vi "Simple_Example_Soft_Trigger.vi"() -> ()   [LabVIEW 2019]
doc: "This example shows a simple recording of an image sequence and the image access afterwards.\nIt is a good starting point for writing own applications.\nBut it will not be fail save, i.e. doesnt react on errors, just handles them forward to the end\n\nUsage:\nSelect your required image count before you start the program. Press the \"Trigger\" button to acquire an image. Once started, the camera class will be initialized and images will be recorded automatically.\nWhen acquisition has finished you can address the images and set a certain roi \nTo finish the program click on quit application, this will force fan exit of the camera class"
uses:
  camera/Camera.lvclass
  <vilib>/picture/picture.llb/Draw 8-Bit Pixmap.vi
  <vilib>/picture/picture.llb/Draw True-Color Pixmap.vi
  pco.sdk/TimingControl/TimingControl.lvlib
panel:
  in  "Trigger":bool
  out "colormap(U8)":u32[](array[numeric])
  out "Image(U16)":u16[][](graph)
  in  "Zoom [%]":i32(slide)=26 min=10 max=200 step=5 scale=10.0..200.0
  out "Image":picture
  out "rawImage":u16[][](array[numeric])
  in  "data_format":T1(ring)=enum."Mono16"
  in  "Image Index":u32 max=9
  out "Recorded Images":u32
  in  "Quit":bool
  in  "cropY1":u64=2 min=2 max=2048 step=1
  in  "cropX1":u64=2 min=2 max=2048 step=1
  in  "cropY0":u64=1 min=1 max=2047 step=1
  in  "cropX0":u64=1 min=1 max=2047 step=1
  out "Image Height":u16
  out "Image Width":u16
  in  "dwImgCount":u32=10 caption="Required Number of Images" max=4023
  out "Error":errorcluster {"code" format="%x"}
  # "This example shows a simple recording of an image sequence using software triggering and the image access afterwards.\nIt is a good starting point for writing own applications.\nBut it will not be fail save, i.e. doesnt react on errors, just handles them forward to the end\n\nUsage:\nSelect your required image count before you start the program. Once started, the camera class will be initialized and images will be recorded automatically. Press the \"Trigger\" button to acquire an image. When acquisition has finished you can address the images and crop them to a smaller size. To finish the program click on quit application, this will force fan exit of the camera class"
  # "pco.labview"
  # "Camera Setup"
  # "Recording Control"
  # "Parameters for image readout"
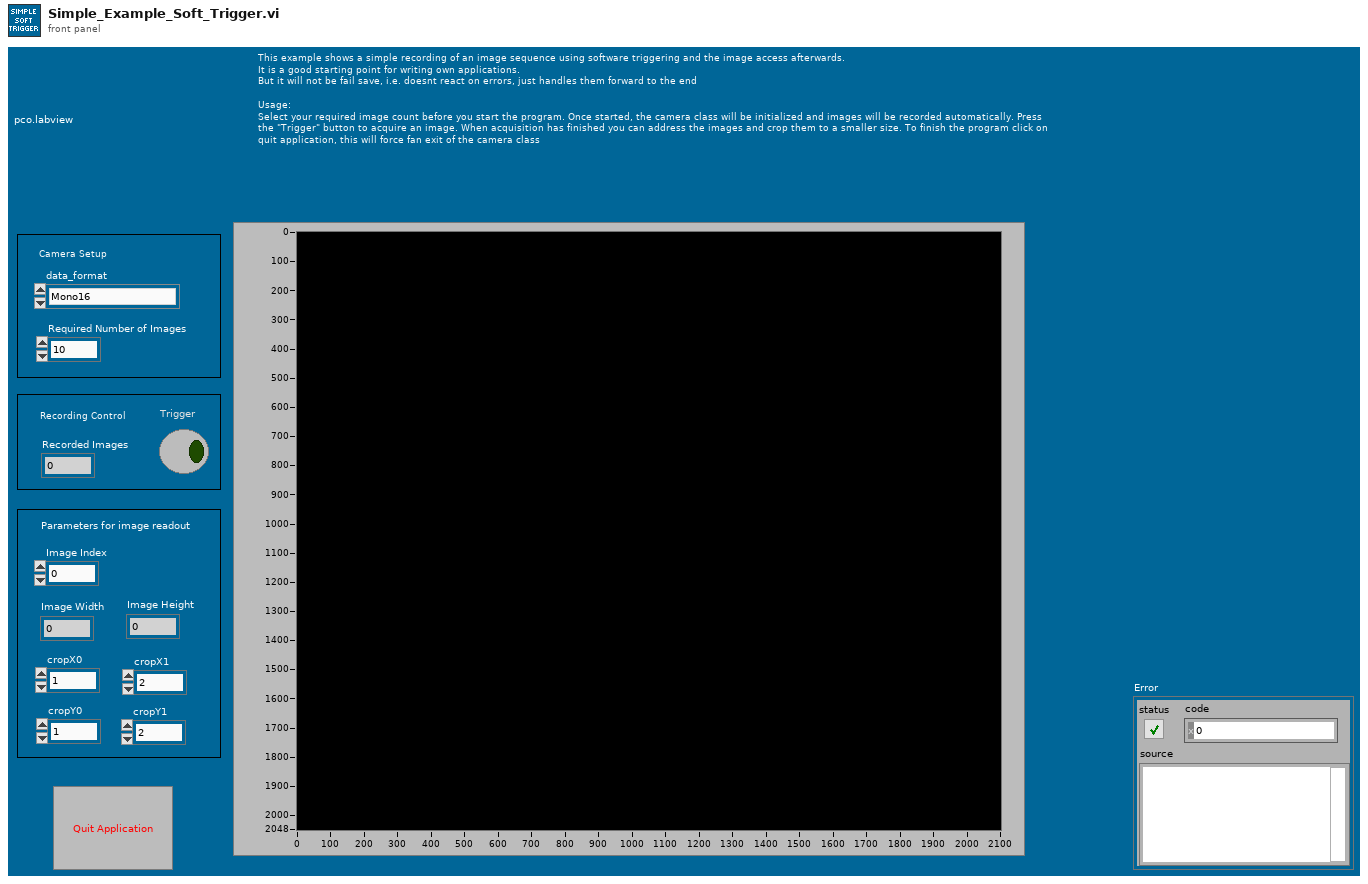
[diagram p1: front panel]
types:
  T1 = enum16{"Undefined", "Mono8", "Mono16", "BGRA8", "RGBA8", "BGRA16", "RGBA16", "CompressedMono8"}
  T2 = enum8{"Enabled", "Disabled", "Disabled and Grayed Out"}
  T3 = enum16{"sequence", "sequence non blocking", "ring buffer", "fifo", "tif", "multitif", "pcoraw", "b16", "dicom", "multidicom", "camram_ring", "camram_segment"}
  T4 = typedef "Camera.lvclass/binning.ctl" = cluster{"vert":u16, "horz":u16, "mode":u16}
  T5 = cluster{"exposure_time_s":dbl, "delay_time_s":dbl, "roi":cluster{"x0":u64, "y0":u64, "x1":u64, "y1":u64}, "timestamp_mode":u16, "pixelrate":u32, "conversion_factor":sgl, "trigger_mode":u16, "acquire_mode":u16, "acquire_sequence_number":u32, "metadata_mode":u16, "noisefilter_mode":u16, "pixel_format":u32, "binning":T4, "auto_exposure":cluster{"region":u16, "min_exposure_s":dbl, "max_exposure_s":dbl}}
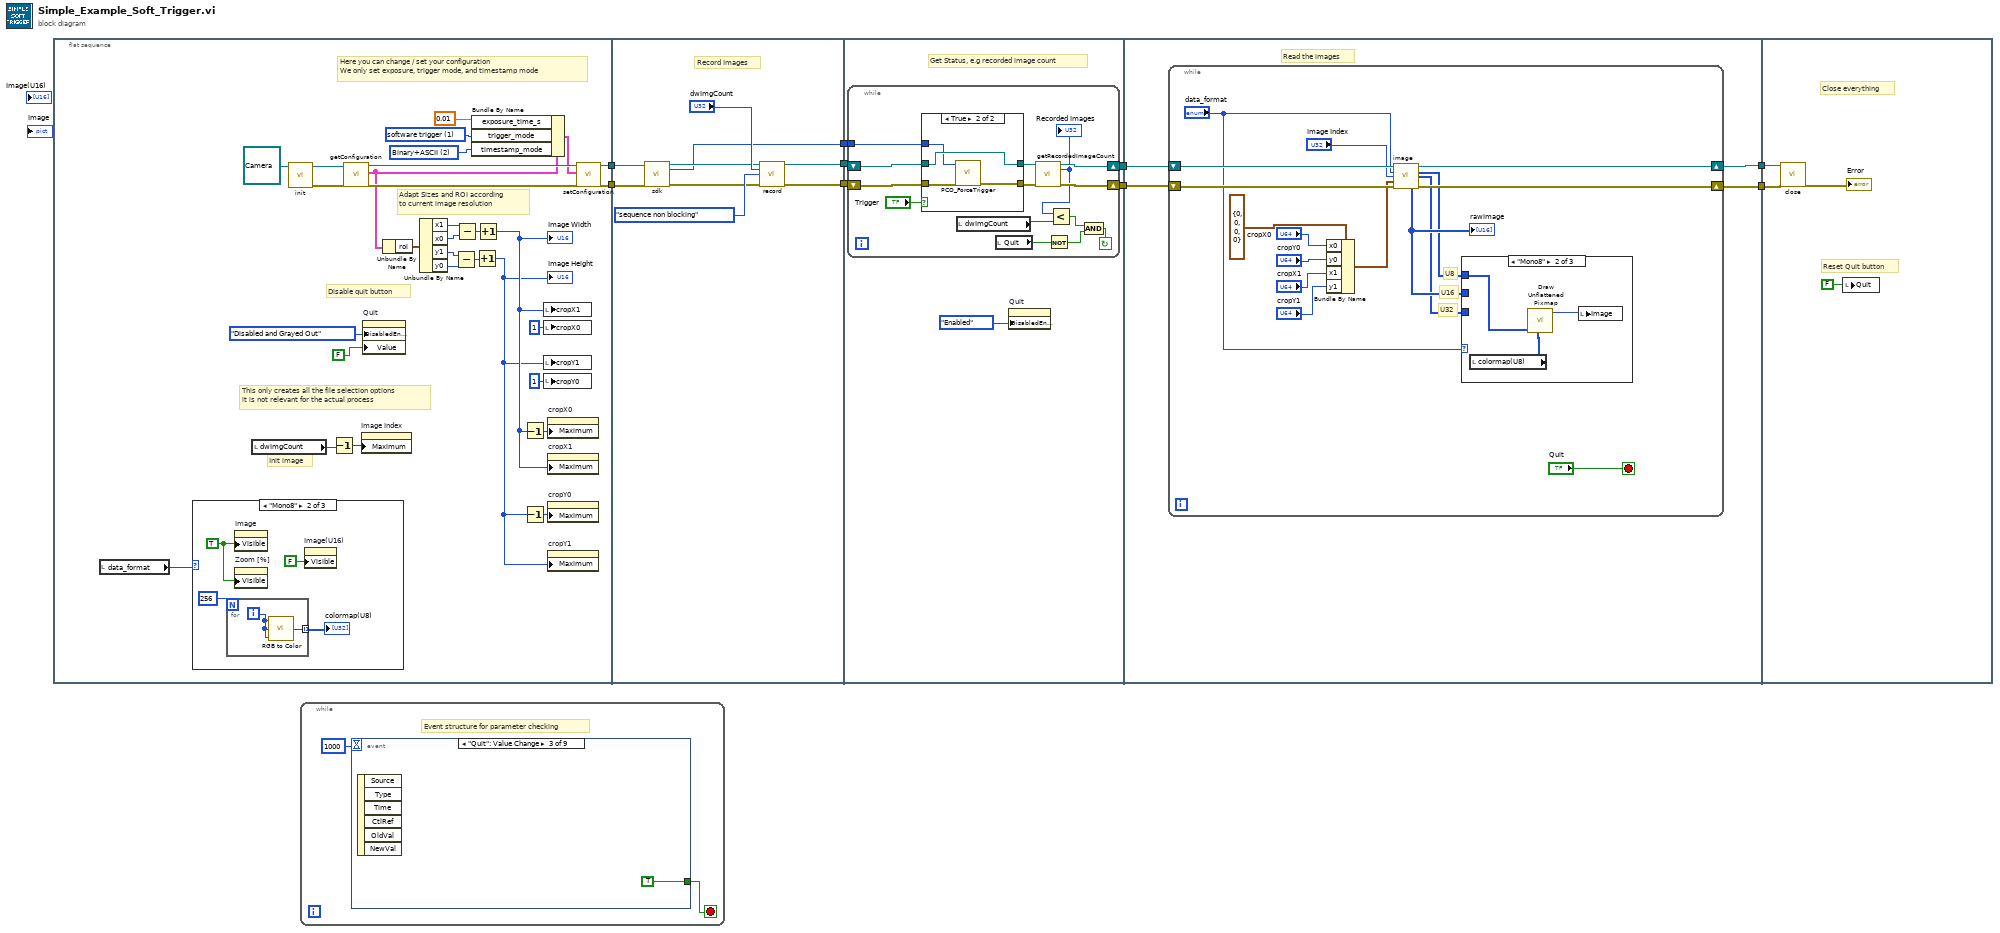
[diagram p0: block diagram]
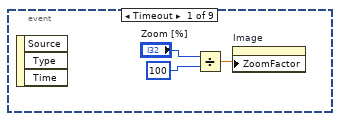
[diagram p2: hidden frame]
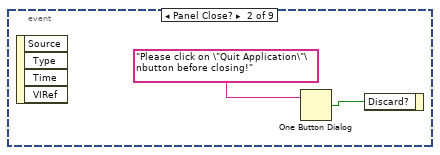
[diagram p3: hidden frame]
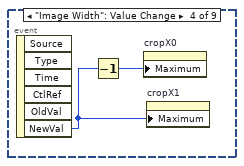
[diagram p4: hidden frame]
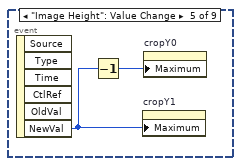
[diagram p5: hidden frame]
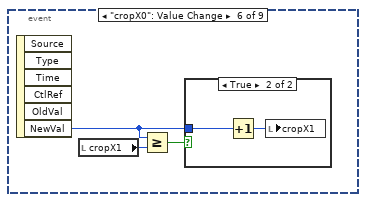
[diagram p6: hidden frame]
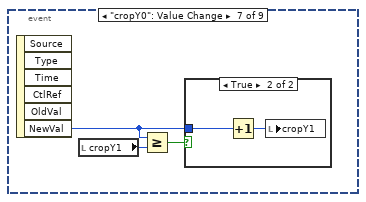
[diagram p8: hidden frame]
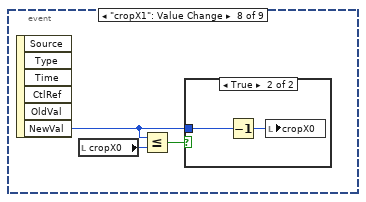
[diagram p10: hidden frame]
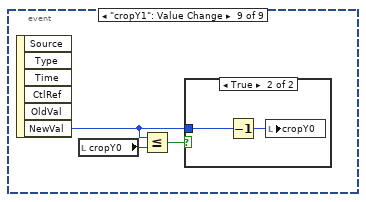
[diagram p12: hidden frame]
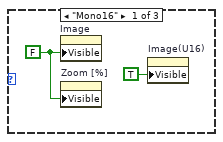
[diagram p14: hidden frame]
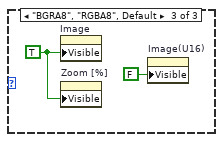
[diagram p15: hidden frame]
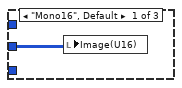
[diagram p17: hidden frame]
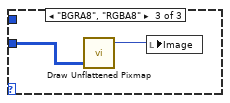
[diagram p18: hidden frame]
diagram:
  n1 = flat-sequence {
    tunnel: [w32] -> w9
    tunnel: [w31] -> w8
    tunnel: w9 -> [w54]
    tunnel: w8 -> [w52]
    tunnel: [w57] -> w7
    tunnel: [w56] -> w6
    tunnel: [w50] -> w1
    tunnel: w7 -> [w61]
    tunnel: w6 -> [w60]
    tunnel: [w64] -> w5
    tunnel: [w63] -> w4
    tunnel: w1 -> [w59]
    tunnel: w5 -> [w87]
    tunnel: w4 -> [w88]
    tunnel: [w86] -> w3
    tunnel: [w85] -> w2
    tunnel: w3 -> [w112]
    tunnel: w2 -> [w111]
    frame #0 {
      w16 = u16 2 items=["OFF", "Binary", "Binary+ASCII", "ASCII"] ("TimestampMode")
      w36 = u16 1 items=["auto sequence"=0, "software trigger"=1, "external exposure start & software trigger"=2, "external exposure control"=3, "external synchronized"=4, "fast external exposure control"=5, "external CDS control"=6, "slow external exposure control"=7, "external synchronized HDSDI"=258] ("TriggerMode")
      # "Here you can change / set your configuration\nWe only set exposure, trigger mode, and timestamp mode"
      # "Init image"
      # "This only creates all the file selection options\nit is not relevant for the actual process"
      # "Adapt Sizes and ROI according\nto current image resolution"
      # "Disable quit button"
      n2 = local read "data_format"() -> (w11:T1)
      n3 = case shown="\"Mono8\"" w11 {
        frame "Mono16" {
          w41 = FALSE ("Visible")
          n4 = property on="Image" class="Pict"("Visible"=w41) -> ()  [unwired: 2 in, 2 out]
          n5 = property on="Zoom [%]" class="Slide (strict)"("Visible"=w41) -> ()  [unwired: 2 in, 2 out]
          n6 = property on="Image(U16)" class="IntGraph (strict)"("Visible"=TRUE) -> ()  [unwired: 2 in, 2 out]
        }
        frame "Mono8" {
          w44 = TRUE ("Visible")
          n7 = for {
            N: 256 -> [_]
            tunnel: [w46] -> w43 mode=indexing
            i -> [w47]
            n8 = call <vilib>:"RGB to Color.vi"("B"=w47, "G"=w47, "R"=w47) -> ("Color"=w46:u32)
          }
          "colormap(U8)" <- w43
          n9 = property on="Image" class="Pict"("Visible"=w44) -> ()  [unwired: 2 in, 2 out]
          n10 = property on="Zoom [%]" class="Slide (strict)"("Visible"=w44) -> ()  [unwired: 2 in, 2 out]
          n11 = property on="Image(U16)" class="IntGraph (strict)"("Visible"=FALSE) -> ()  [unwired: 2 in, 2 out]
        }
        frame "BGRA8", "RGBA8", Default {
          w48 = TRUE ("Visible")
          n12 = property on="Image" class="Pict"("Visible"=w48) -> ()  [unwired: 2 in, 2 out]
          n13 = property on="Zoom [%]" class="Slide (strict)"("Visible"=w48) -> ()  [unwired: 2 in, 2 out]
          n14 = property on="Image(U16)" class="IntGraph (strict)"("Visible"=FALSE) -> ()  [unwired: 2 in, 2 out]
        }
      }
      n15 = local read "dwImgCount"() -> (w12:u32)
      n16 = call-dynamic "init.vi"("Camera in"=refnum<class "Camera.lvclass"> refnum ("PCOCamera in")) -> ("Camera out"=w38:refnum<class "Camera.lvclass">, "error out"=w37:errorcluster)  [unwired: 8 in]
      n17 = Decrement(x=w12) -> (x-1=w13:u32)
      n18 = call-dynamic "getConfiguration.vi"("error in (no error)"=w37, "Camera in"=w38) -> ("error out"=w34:errorcluster, "configuration"=w26:T5, "Camera out"=w35:refnum<class "Camera.lvclass">)  [unwired: 7 in]
      n19 = property on="Image Index" class="DigNum (strict)"("Maximum"=w13) -> ()  [unwired: 2 in, 2 out]
      n20 = property on="Quit" class="Bool (strict)"("DisabledEnum"=T2."Disabled and Grayed Out" ("Disabled"), "Value"=FALSE ("Stop")) -> ()  [unwired: 2 in, 2 out]
      n21 = Unbundle By Name(w26) -> ("roi"=w25:cluster{"x0":u64, "y0":u64, "x1":u64, "y1":u64})
      n22 = Unbundle By Name(w25) -> ("x1"=w23:u64, "x0"=w24:u64, "y1"=w21:u64, "y0"=w22:u64)
      n23 = Subtract(x=w21, y=w22) -> (x-y=w19:u64)
      n24 = Subtract(x=w23, y=w24) -> (x-y=w20:u64)
      n25 = Bundle By Name(cluster=w26, "exposure_time_s"=0.01, "trigger_mode"=w36, "timestamp_mode"=w16) -> (w33:T5)
      n26 = Increment(x=w19) -> (x+1=w17:u64)
      "Image Height" <- w17
      n27 = Increment(x=w20) -> (x+1=w18:u64)
      "Image Width" <- w18
      n28 = Decrement(x=w18) -> (x-1=w28:u64)
      n29 = Decrement(x=w17) -> (x-1=w27:u64)
      n30 = local write "cropX1"(w18) -> ()
      n31 = local write "cropX0"(u16 1 ("roiY0")) -> ()
      n32 = local write "cropY1"(w17) -> ()
      n33 = local write "cropY0"(u16 1 ("roiY0")) -> ()
      n34 = property on="cropX0" class="DigNum (strict)"("Maximum"=w28) -> ()  [unwired: 2 in, 2 out]
      n35 = property on="cropX1" class="DigNum (strict)"("Maximum"=w18) -> ()  [unwired: 2 in, 2 out]
      n36 = property on="cropY0" class="DigNum (strict)"("Maximum"=w27) -> ()  [unwired: 2 in, 2 out]
      n37 = property on="cropY1" class="DigNum (strict)"("Maximum"=w17) -> ()  [unwired: 2 in, 2 out]
      n38 = call-dynamic "setConfiguration.vi"("error in (no error)"=w34, "configuration"=w33, "Camera in"=w35) -> ("error out"=w31:errorcluster, "Camera out"=w32:refnum<class "Camera.lvclass">)  [unwired: 7 in]
    }
    frame #1 {
      # "Record Images"
      n39 = call-dynamic "sdk.vi"("Camera in"=w54, "error in (no error)"=w52) -> ("Camera out"=w53:refnum<class "Camera.lvclass">, "sdk"=w50:u64, "error out"=w51:errorcluster)  [unwired: 11 in]
      n40 = call-dynamic "record.vi"("Camera in"=w53, "num_images"="dwImgCount", "record_mode"=T3."sequence non blocking", "error in (no error)"=w51) -> ("Camera out"=w57:refnum<class "Camera.lvclass">, "error out"=w56:errorcluster)  [unwired: 10 in]
    }
    frame #2 {
      # "Get Status, e.g recorded image count"
      n41 = while {
        tunnel: w59 -> [w72]
        shift-right: [w78] -> w64
        shift-left: w61 -> [w76]
        shift-right: [w77] -> w63
        shift-left: w60 -> [w74]
        stop <- w65 continue-if-true
        n42 = case shown="True" "Trigger" {
          tunnel: w76 -> [w80 w84]
          tunnel: [w80 w84] -> w75
          tunnel: w74 -> [w79 w83]
          tunnel: [w79 w82] -> w73
          tunnel: w72 -> [_ w81]
          frame False {
          }
          frame True {
            n43 = call "PCO_ForceTrigger.vi"("error in (no error)"=w83, "ph"=w81) -> ("error out"=w82:errorcluster)  [unwired: 6 in, 3 out]
          }
        }
        n44 = local read "dwImgCount"() -> (w70:u32)
        n45 = local read "Quit"() -> (w68:bool)
        n46 = call-dynamic "getRecordedImageCount.vi"("Camera in"=w75, "error in (no error)"=w73) -> ("Camera out"=w78:refnum<class "Camera.lvclass">, "recorded_image_count"=w69:u32, "error out"=w77:errorcluster)  [unwired: 11 in]
        "Recorded Images" <- w69
        n47 = Not(x=w68) -> (.not. x?=w67:bool)
        n48 = Less?(x=w69, y=w70) -> (x < y?=w66:bool)
        n49 = And(x=w66, y=w67) -> (x .and. y?=w65:bool)
      }
      n50 = property on="Quit" class="Bool (strict)"("DisabledEnum"=T2."Enabled" ("Disabled")) -> ()  [unwired: 2 in, 2 out]
    }
    frame #3 {
      # "Read the images"
      n51 = while {
        shift-right: [w102] -> w86
        shift-left: w87 -> [w104]
        shift-right: [w97] -> w85
        shift-left: w88 -> [w103]
        stop <- "Quit" stop-if-true
        # "U32"
        # "U16"
        # "U8"
        n52 = Bundle By Name(cluster=cluster{"x0":u64, "y0":u64, "x1":u64, "y1":u64} {"x0"=0, "y0"=0, "x1"=0, "y1"=0} ("roi"), "x0"="cropX0", "y0"="cropY0", "x1"="cropX1", "y1"="cropY1") -> (w96:cluster{"x0":u64, "y0":u64, "x1":u64, "y1":u64})
        n53 = call-dynamic "image.vi"("Camera in"=w104, "data_format"="data_format", "image_index"="Image Index", "crop"=w96, "error in (no error)"=w103) -> ("Camera out"=w102:refnum<class "Camera.lvclass">, "image (U8)"=w89:u8[][], "image (U32)"=w90:u32[][], "raw_image (U16)"=w91:u16[][], "error out"=w97:errorcluster)  [unwired: 2 in, 4 out]
        "rawImage" <- w91
        n54 = case shown="\"Mono8\"" "data_format" {
          tunnel: w90 -> [_ _ w110]
          tunnel: w89 -> [_ w107 _]
          tunnel: w91 -> [w105 _ _]
          frame "Mono16", Default {
            n55 = local write "Image(U16)"(w105) -> ()
          }
          frame "Mono8" {
            n56 = local read "colormap(U8)"() -> (w106:u32[])
            n57 = call-poly <vilib>:"Draw Unflattened Pixmap.vi"("data"=w107, "color table"=w106) -> ("new picture"=w108:picture)  [unwired: 7 in]
            n58 = local write "Image"(w108) -> ()
          }
          frame "BGRA8", "RGBA8" {
            n59 = call-poly <vilib>:"Draw Unflattened Pixmap.vi"("data (RGB format)"=w110) -> ("new picture"=w109:picture)  [unwired: 8 in]
            n60 = local write "Image"(w109) -> ()
          }
        }
      }
    }
    frame #4 {
      # "Reset Quit button"
      # "Close everything"
      n61 = call-dynamic "close.vi"("error in (no error)"=w111, "Camera in"=w112) -> ("error out"=→"Error":errorcluster)  [unwired: 9 in]
      n62 = local write "Quit"(FALSE ("Stop")) -> ()
    }
  }
  n63 = while {
    stop <- w115 stop-if-true
    # "Event structure for parameter checking"
    n64 = event shown="[2] \"Quit\": Value Change" {
      selector: _ -> [_ _ _ _ _ _ _ _ _]
      dyn-events: _ -> [_ _ _ _ _ _ _ _ _]
      timeout: 1000 -> [_ _ _ _ _ _ _ _ _]
      tunnel: [_ _ TRUE _ _ _ _ _ _] -> w115
      event Timeout {
        n65 = event-data() -> ()  [unwired: 1 in, 3 out]
        n66 = Divide(x="Zoom [%]", y=100 ("Zoom [%]")) -> (x/y=w117:dbl)
        n67 = property on="Image" class="Pict"("ZoomFactor"=w117) -> ()  [unwired: 2 in, 2 out]
      }
      event Panel Close? {
        n68 = event-data() -> ()  [unwired: 1 in, 4 out]
        n69 = One Button Dialog(message="Please click on \"Quit Application\"\nbutton before closing!") -> (true=w120:bool)  [unwired: 1 in]
        n70 = event-data("Discard?"=w120) -> ()  [unwired: 1 in, 1 out]
      }
      event "Quit": Value Change {
        n71 = event-data() -> ()  [unwired: 1 in, 6 out]
      }
      event "Image Width": Value Change {
        n72 = event-data() -> ("NewVal"=w123:u16)  [unwired: 1 in, 5 out]
        n73 = Decrement(x=w123) -> (x-1=w124:u16)
        n74 = property on="cropX0" class="DigNum (strict)"("Maximum"=w124) -> ()  [unwired: 2 in, 2 out]
        n75 = property on="cropX1" class="DigNum (strict)"("Maximum"=w123) -> ()  [unwired: 2 in, 2 out]
      }
      event "Image Height": Value Change {
        n76 = event-data() -> ("NewVal"=w125:u16)  [unwired: 1 in, 5 out]
        n77 = Decrement(x=w125) -> (x-1=w126:u16)
        n78 = property on="cropY1" class="DigNum (strict)"("Maximum"=w125) -> ()  [unwired: 2 in, 2 out]
        n79 = property on="cropY0" class="DigNum (strict)"("Maximum"=w126) -> ()  [unwired: 2 in, 2 out]
      }
      event "cropX0": Value Change {
        n80 = event-data() -> ("NewVal"=w127:u64)  [unwired: 1 in, 5 out]
        n81 = local read "cropX1"() -> (w129:u64)
        n82 = Greater Or Equal?(x=w127, y=w129) -> (x >= y?=w128:bool)
        n83 = case shown="True" w128 {
          tunnel: w127 -> [_ w131]
          frame False {
          }
          frame True {
            n84 = Increment(x=w131) -> (x+1=w130:u64)
            n85 = local write "cropX1"(w130) -> ()
          }
        }
      }
      event "cropY0": Value Change {
        n86 = event-data() -> ("NewVal"=w132:u64)  [unwired: 1 in, 5 out]
        n87 = local read "cropY1"() -> (w134:u64)
        n88 = Greater Or Equal?(x=w132, y=w134) -> (x >= y?=w133:bool)
        n89 = case shown="True" w133 {
          tunnel: w132 -> [_ w136]
          frame False {
          }
          frame True {
            n90 = Increment(x=w136) -> (x+1=w135:u64)
            n91 = local write "cropY1"(w135) -> ()
          }
        }
      }
      event "cropX1": Value Change {
        n92 = event-data() -> ("NewVal"=w137:u64)  [unwired: 1 in, 5 out]
        n93 = local read "cropX0"() -> (w139:u64)
        n94 = Less Or Equal?(x=w137, y=w139) -> (x <= y?=w138:bool)
        n95 = case shown="True" w138 {
          tunnel: w137 -> [_ w141]
          frame False {
          }
          frame True {
            n96 = Decrement(x=w141) -> (x-1=w140:u64)
            n97 = local write "cropX0"(w140) -> ()
          }
        }
      }
      event "cropY1": Value Change {
        n98 = event-data() -> ("NewVal"=w142:u64)  [unwired: 1 in, 5 out]
        n99 = local read "cropY0"() -> (w144:u64)
        n100 = Less Or Equal?(x=w142, y=w144) -> (x <= y?=w143:bool)
        n101 = case shown="True" w143 {
          tunnel: w142 -> [_ w146]
          frame False {
          }
          frame True {
            n102 = Decrement(x=w146) -> (x-1=w145:u64)
            n103 = local write "cropY0"(w145) -> ()
          }
        }
      }
    }
  }
